vi "sendValue.vi"(8 "error in (no error)":errorcluster, 10 "data":variant, 11 "rejectedCommand in":refnum<class "rejectedCommand.lvclass">) -> (0 "error out":errorcluster, 2 "function return":i32, 3 "rejectedCommand out":refnum<class "rejectedCommand.lvclass">)   [LabVIEW 2016, in "SALLV_MtAtElectrometer_Messaging.lvlib" / "rejectedCommand.lvclass"]
uses:
  rejectedCommand.lvclass
  ts_sallv_MtAtElectrometer/DataTypes/logevent_rejectedCommand.ctl
  ts_sallv_MtAtElectrometer/SALLV_MtAtElectrometer.lvlib
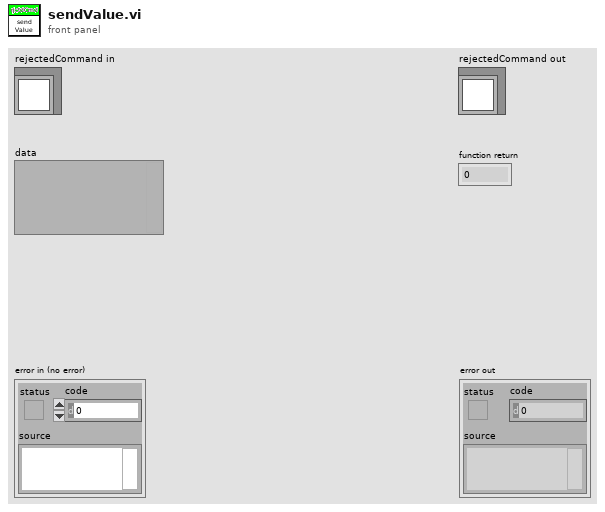
[diagram p1: front panel]
types:
  T1 = typedef "SALLV_MtAtElectrometer.lvlib/logevent_rejectedCommand.ctl" = cluster{"commandValue":u16, "detailedState":u16, "timestamp":dbl, "priority":i32}
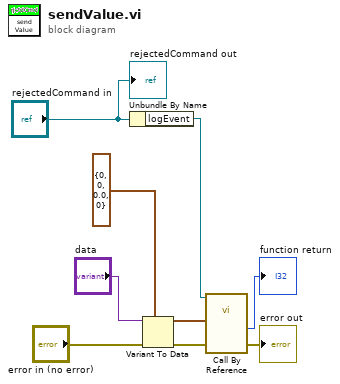
[diagram p0: block diagram]
diagram:
  n1 = Unbundle By Name("rejectedCommand in") -> ("logEvent"=w7:refnum<vi>)
  n2 = Variant To Data(error in="error in (no error)", type=T1 {"commandValue"=0, "detailedState"=0, "timestamp"=0.0, "priority"=0} ("logevent_rejectedCommand"), Variant="data") -> (data=w1:T1, error out=w5:errorcluster)
  n3 = call-by-ref "?"(reference=w7, "error in (no error)"=w5, "logevent_rejectedCommand_Ctl"=w1) -> ("error out"=→"error out":errorcluster, "function return"=→"function return":i32)  [unwired: 8 in, 3 out]
  "rejectedCommand out" <- "rejectedCommand in"
